vi "Set Temp Ramp Rate--Method.vi"(8 "error in (no error)":errorcluster, 10 "Temp Ramp Data":T1, 11 "_Thermal Process Controller in":refnum<class "_Thermal Process Controller.lvclass">) -> (0 "error out":errorcluster, 3 "_Thermal Process Controller out":refnum<class "_Thermal Process Controller.lvclass">)   [LabVIEW 2024, in "_Thermal Process Controller.lvclass"]
uses:
  _Thermal Process Controller.lvclass
  Controls/Temp Ramp Rate Data--Cluster.ctl
  Controls/Temperature Units--Enum.ctl
  Controls/Rate Units--Enum.ctl
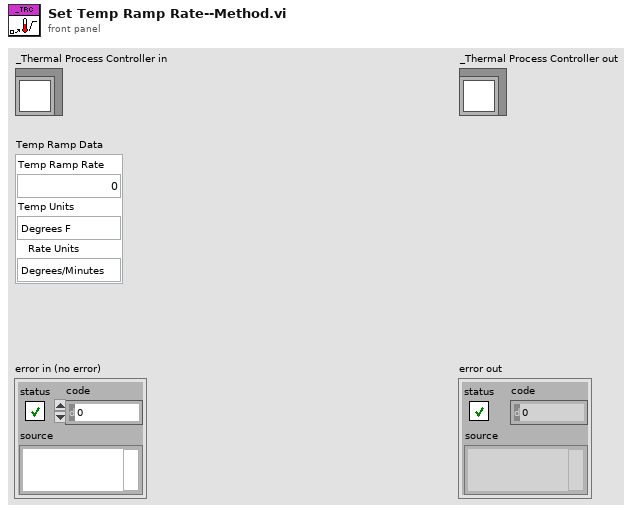
[diagram p1: front panel]
types:
  T1 = typedef "_Thermal Process Controller.lvclass/Temp Ramp Rate Data--Cluster.ctl" = cluster{"Temp Ramp Rate":dbl, "Temp Units":T2, "Rate Units":T3}
  T2 = typedef "_Thermal Process Controller.lvclass/Temperature Units--Enum.ctl" = enum16{"Degrees F", "Degrees C", "Degrees K"}
  T3 = typedef "_Thermal Process Controller.lvclass/Rate Units--Enum.ctl" = enum16{"Degrees/Minutes", "Degrees/Hours"}
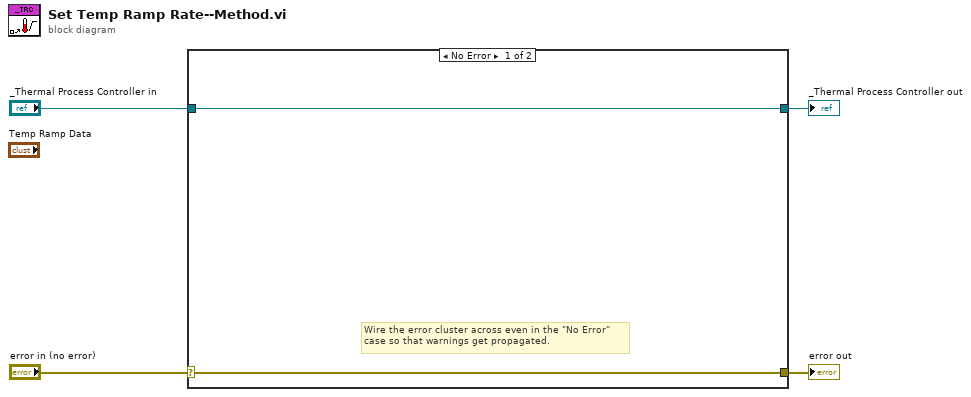
[diagram p0: block diagram]
diagram:
  n1 = case shown="No Error" "error in (no error)" {
    selector: "error in (no error)" -> [w5 w8]
    tunnel: [w5 w8] -> w3
    tunnel: [w6 w7] -> w1
    tunnel: "_Thermal Process Controller in" -> [w6 w7]
    frame No Error {
      # "Wire the error cluster across even in the \"No Error\"\ncase so that warnings get propagated."
    }
    frame Error {
    }
  }
  "error out" <- w3
  "_Thermal Process Controller out" <- w1
